vi "ReceiveStringMessage.vi"(8 "error in (no error)":errorcluster, 11 "TCP_Server_Connection_Handler in":refnum<class "TCP_Server_Connection_Handler.lvclass">) -> (0 "error out":errorcluster, 2 "message out":string, 3 "TCP_Server_Connection_Handler out":refnum<class "TCP_Server_Connection_Handler.lvclass">)   [LabVIEW 2023]
uses:
  TCP_Server_Connection_Handler.lvclass
  C:/Program Files (x86)/National Instruments/LabVIEW 2023/vi.lib/ActorFramework/Actor/Actor.lvclass
  TypeDefinitions/ClientMessage.ctl
  TCP_Server_Connection_Handler.lvclass/TCP_Server_Connection_Handler.ctl
  <vilib>/ActorFramework/Actor/Actor.lvclass/Actor.ctl
  <vilib>/ActorFramework/Message Enqueuer/Message Enqueuer.lvclass/Message Enqueuer.ctl
  TCP_Connections_Controller Messages/MessageRecieved Msg/MessageRecieved Msg.lvclass/MessageRecieved Msg.ctl
  <vilib>/ActorFramework/Message Enqueuer/Init from Existing Queue.vi
  <vilib>/ActorFramework/Message Enqueuer/Enqueue.vi
  TCP_Server_Connection_Handler Messages/FindMessageStart Msg/FindMessageStart Msg.lvclass
  C:/Program Files (x86)/National Instruments/LabVIEW 2023/vi.lib/ActorFramework/Message/Message.lvclass
  TCP_Connections_Controller Messages/MessageRecieved Msg/MessageRecieved Msg.lvclass
  <vilib>/ActorFramework/Message Priority Queue/Priority Enqueue.vi
  <vilib>/ActorFramework/Message Enqueuer/Message Enqueuer.lvclass
  <vilib>/ActorFramework/Actor/Actor.lvclass
  TCP_Server_Connection_Handler.lvlib
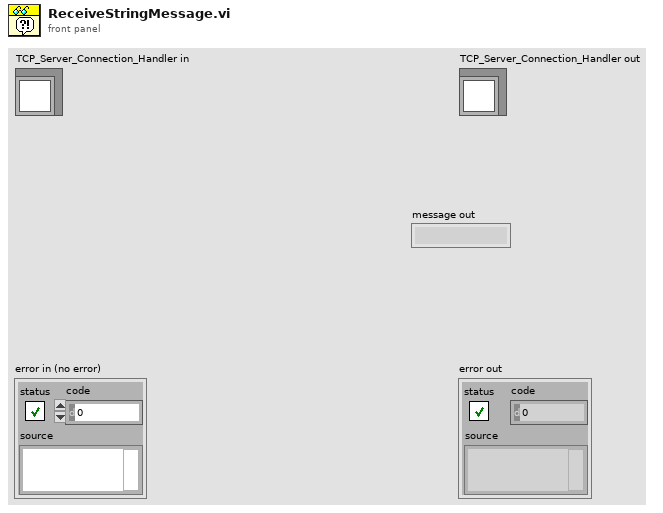
[diagram p1: front panel]
types:
  T1 = typedef "TCP_Server_Connection_Handler.lvlib/ClientMessage.ctl" = cluster{"ConnectionNumber":i32, "ClientIP":string, "Message":string}
  T2 = typedef "TCP_Listener.lvlib/ConnectionInformation.ctl" = cluster{"Connection number":i32, "Remote Address":string, "Remote Port":u16, "Connection ID":refnum<k5>}
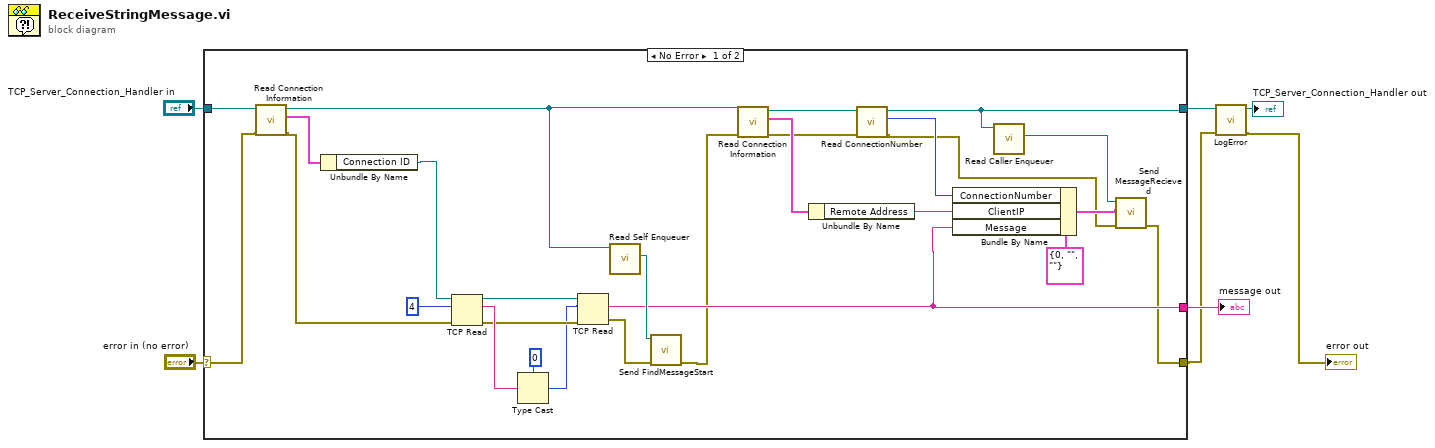
[diagram p0: block diagram]
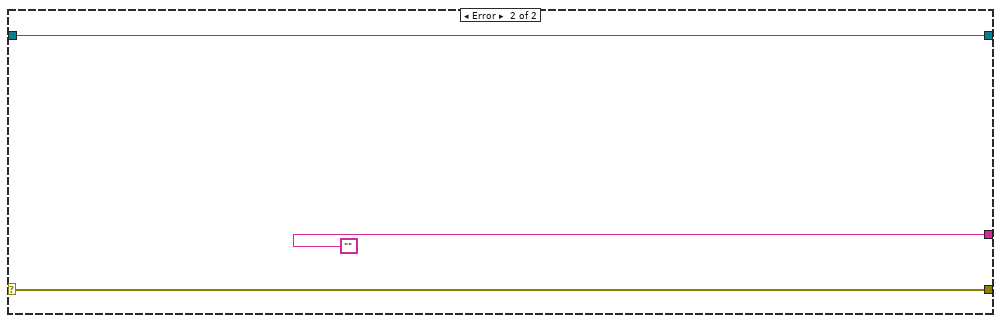
[diagram p2: hidden frame]
diagram:
  n1 = case shown="No Error" "error in (no error)" {
    selector: "error in (no error)" -> [w25 w37]
    tunnel: [w8 w37] -> w2
    tunnel: [w19 w36] -> w4
    tunnel: "TCP_Server_Connection_Handler in" -> [w34 w36]
    tunnel: [w14 ""] -> w5
    frame No Error {
      n2 = call "Read Connection Information.vi"("error in (no error)"=w25, "TCP_Server_Connection_Handler in"=w34) -> ("error out"=w24:errorcluster, "Connection Information"=w33:T2, "TCP_Server_Connection_Handler out"=w21:refnum<class "TCP_Server_Connection_Handler.lvclass">)  [unwired: 7 in]
      n3 = Unbundle By Name(w33) -> ("Connection ID"=w32:refnum<k5>)
      n4 = TCP Read(connection ID=w32, bytes to read=4, error in (no error)=w24) -> (connection ID out=w28:refnum<k5>, data out=w30:string, error out=w27:errorcluster)  [unwired: 2 in]
      n5 = Type Cast(type=0, x=w30) -> (*(type *) &x=w26:i32)
      n6 = TCP Read(connection ID=w28, bytes to read=w26, error in (no error)=w27) -> (data out=w14:string, error out=w22:errorcluster)  [unwired: 2 in, 1 out]
      n7 = call <vilib>:"Read Self Enqueuer.vi"("Actor"=w21) -> ("Self Enqueuer"=w23:refnum<class "Message Enqueuer.lvclass">)  [unwired: 10 in]
      n8 = call "Send FindMessageStart.vi"("error in (no error)"=w22, "Message Enqueuer"=w23) -> ("error out"=w11:errorcluster)  [unwired: 8 in, 1 out]
      n9 = call "Read Connection Information.vi"("error in (no error)"=w11, "TCP_Server_Connection_Handler in"=w21) -> ("error out"=w10:errorcluster, "Connection Information"=w13:T2, "TCP_Server_Connection_Handler out"=w20:refnum<class "TCP_Server_Connection_Handler.lvclass">)  [unwired: 7 in]
      n10 = Unbundle By Name(w13) -> ("Remote Address"=w12:string)
      n11 = call "Read ConnectionNumber.vi"("error in (no error)"=w10, "TCP_Server_Connection_Handler in"=w20) -> ("error out"=w9:errorcluster, "ConnectionNumber"=w16:i32, "TCP_Server_Connection_Handler out"=w19:refnum<class "TCP_Server_Connection_Handler.lvclass">)  [unwired: 7 in]
      n12 = Bundle By Name(cluster=T1 {"ConnectionNumber"=0, "ClientIP"="", "Message"=""} ("clientMessage"), "ConnectionNumber"=w16, "ClientIP"=w12, "Message"=w14) -> (w15:T1)
      n13 = call <vilib>:"Read Caller Enqueuer.vi"("Actor"=w19) -> ("Caller Enqueuer"=w18:refnum<class "Message Enqueuer.lvclass">)  [unwired: 10 in]
      n14 = call "Send MessageRecieved.vi"("error in (no error)"=w9, "clientMessage"=w15, "Message Enqueuer"=w18) -> ("error out"=w8:errorcluster)  [unwired: 7 in, 1 out]
    }
    frame Error {
    }
  }
  "message out" <- w5
  n15 = call "LogError.vi"("error in (no error)"=w2, "TCP_Server_Connection_Handler in"=w4) -> ("error out"=→"error out":errorcluster, "TCP_Server_Connection_Handler out"=→"TCP_Server_Connection_Handler out":refnum<class "TCP_Server_Connection_Handler.lvclass">)  [unwired: 8 in]
